vi "Set XY plot from array (subVi).vi"(2 "Average array":dbl[][](array[numeric]), 3 "Spectrum_plot":refnum<vi>) -> (0 "XY Graph":cluster{"X":dbl, "Y":dbl}[](graph))   [LabVIEW 2016]
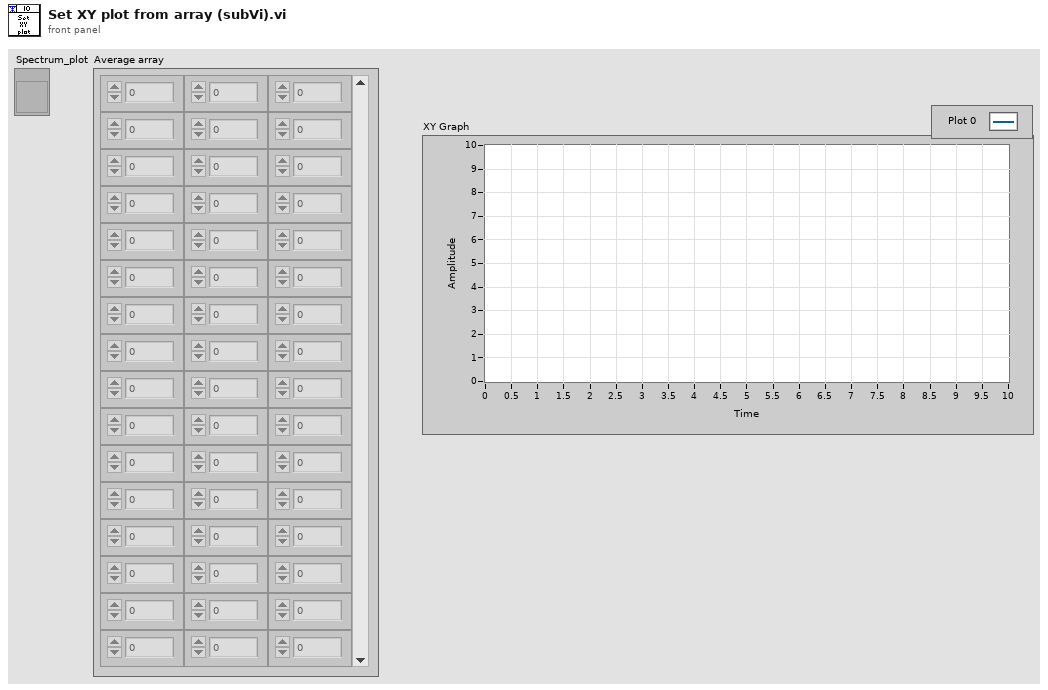
[diagram p1: front panel]
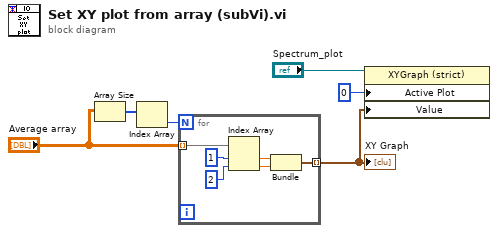
[diagram p0: block diagram]
diagram:
  n1 = Array Size(array="Average array") -> (size(s)=w6:i32[])
  n2 = Index Array(array=w6) -> (element=w5:i32)  [unwired: 1 in]
  n3 = for {
    N: w5 -> [_]
    tunnel: "Average array" -> [w10] mode=indexing
    tunnel: [w7] -> w1 mode=indexing
    n4 = Index Array(array=w10, index #1=1 ("index"), index #2=2 ("index")) -> (element #1=w9:dbl, element #2=w8:dbl)
    n5 = Bundle("Numeric"=w9, "Numeric"=w8) -> (w7:cluster{"Numeric":dbl, "Numeric":dbl})  [unwired: 1 in]
  }
  "XY Graph" <- w1
  n6 = property class="XYGraph (strict)"(reference="Spectrum_plot", "Active Plot"=u32 0, "Value"=w1) -> ()  [unwired: 1 in, 2 out]
